vi "Stop Processes.vi"(11 "VS Inline Async API in":refnum<class "VS Inline Async API.lvclass">) -> (3 "VS Inline Async API out":refnum<class "VS Inline Async API.lvclass">)   [LabVIEW 2027, in "VS Inline Async API.lvlib" / "VS Inline Async API.lvclass"]
uses:
  VS Inline Async API.lvclass
  VS Inline Async API.lvclass/VS Inline Async API.ctl
  <vilib>/NI VeriStand/Custom Device Tools/Custom Device Utility Library/Custom Device Utility Library.lvlib
  <vilib>/Utility/SystemLogging/NI_SystemLogging.lvlib
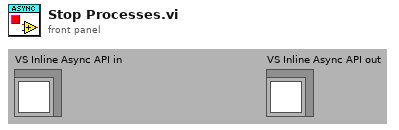
[diagram p1: front panel]
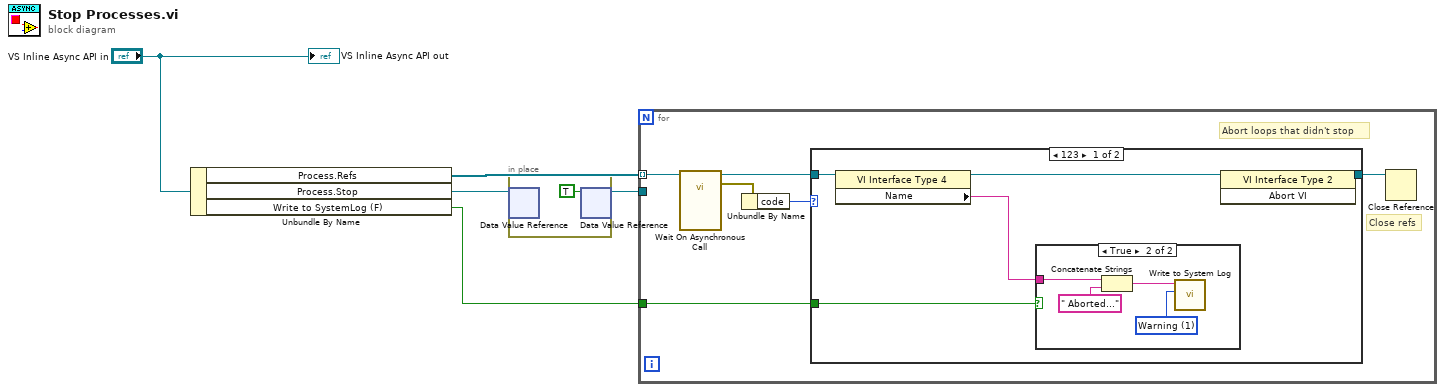
[diagram p0: block diagram]
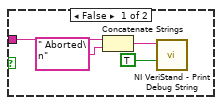
[diagram p2: hidden frame]
diagram:
  n1 = Unbundle By Name("VS Inline Async API in") -> ("Process.Refs"=w3:refnum<vi>[], "Process.Stop"=w4:refnum<data-value>, "Write to SystemLog (F)"=w1:bool)
  n2 = in-place {
    n3 = in-place-dvr #1(w4) -> ()  [unwired: 2 out]
    n4 = in-place-dvr #1(TRUE ("data value")) -> (w2:refnum<data-value>)  [unwired: 1 out]
  }
  n5 = for {
    tunnel: w3 -> [w12] mode=indexing
    tunnel: w2 -> [_]
    tunnel: w1 -> [w7]
    # "Close refs"
    # "Abort loops that didn't stop"
    n6 = call-by-ref "Wait On Asynchronous Call"(reference=w12) -> (reference out=w10:refnum<vi>, error out=w9:errorcluster)  [unwired: 13 in]
    n7 = Unbundle By Name(w9) -> ("code"=w8:i32)
    n8 = case shown="123" w8 {
      tunnel: w10 -> [w16 w26]
      tunnel: [w14 w26] -> w11
      tunnel: w7 -> [w13 _]
      frame 123 {
        n9 = property class="VI Interface Type 4"(reference=w16) -> (reference out=w15:refnum<vi>, "Name"=w17:string)  [unwired: 1 in, 1 out]
        n10 = case shown="True" w13 {
          tunnel: w17 -> [w21 w24]
          frame False {
            n11 = Concatenate Strings(w21, " Aborted\n" ("string")) -> (w19:string)
            n12 = call <vilib>:"NI VeriStand - Print Debug String.vi"("Add to log file? (F)"=TRUE ("Add to log file? (T)"), "Message"=w19) -> ()  [unwired: 9 in, 1 out]
          }
          frame True {
            w22 = 1 items=["Error", "Warning", "Informational"] ("severity")
            n13 = Concatenate Strings(w24, " Aborted..." ("string")) -> (w23:string)
            n14 = call <vilib>:"Write to System Log.vi"("severity"=w22, "message"=w23) -> ()  [unwired: 9 in, 1 out]
          }
        }
        n15 = invoke class="VI Interface Type 2" method="Abort VI"(reference=w15) -> (reference out=w14:refnum<vi>)  [unwired: 2 in, 2 out]
      }
      frame Default {
      }
    }
    n16 = Close Reference(reference=w11) -> ()  [unwired: 1 in, 1 out]
  }
  "VS Inline Async API out" <- "VS Inline Async API in"
